vi "Begin.vi"(8 "error in (no error)":errorcluster, 11 "Blocker in":refnum<class "Blocker.lvclass">) -> (0 "error out":errorcluster, 3 "Blocker out":refnum<class "Blocker.lvclass">)   [LabVIEW 2013, in "Blocker.lvclass"]
uses:
  Blocker.lvclass
  <vilib>/Rock Robotics/WPI/Solenoid/WPI_SolenoidChannel.ctl
  <vilib>/Rock Robotics/SystemInterfaces/Typedef/FPGA_TypedefSolenoidModule.ctl
  System/System.lvclass
  <vilib>/Rock Robotics/WPI/Solenoid/WPI_SolenoidOpenSingle.vi
panel:
  in  "Solenoid Module (Module 1)":T1
  in  "Solenoid Channel":T2=enum."Solenoid 5"
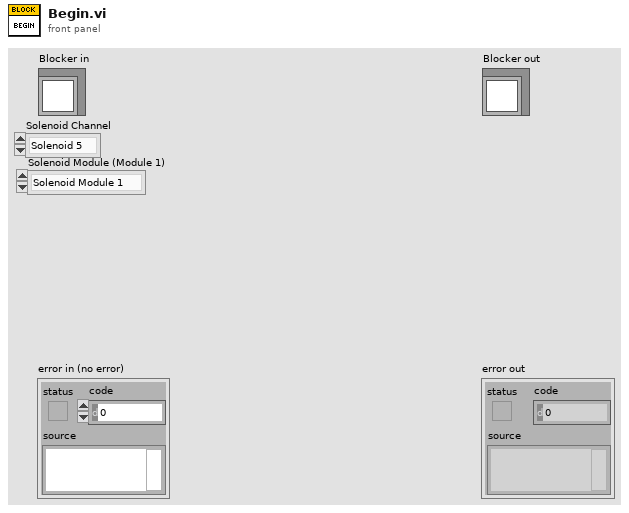
[diagram p1: front panel]
types:
  T1 = typedef "FPGA_TypedefSolenoidModule.ctl" = enum16{"Solenoid Module 1", "Solenoid Module 2"}
  T2 = typedef "WPI_SolenoidChannel.ctl" = enum8{"Solenoid 1", "Solenoid 2", "Solenoid 3", "Solenoid 4", "Solenoid 5", "Solenoid 6", "Solenoid 7", "Solenoid 8", "Invalid"}
  T3 = typedef "WPI_SolenoidDevRef.ctl" = cluster{"DevStatus":errorcluster, "Solenoid Module":T1, "Forward Solenoid Channel":T2, "Reverse Solenoid Channel":T2}
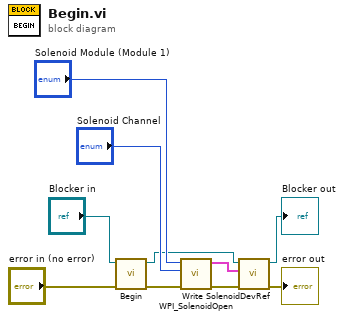
[diagram p0: block diagram]
diagram:
  n1 = call-parent "Begin.vi"("error in (no error)"="error in (no error)", "System in"="Blocker in") -> ("error out"=w2:errorcluster, "System out"=w5:refnum<class "Blocker.lvclass">)  [unwired: 8 in]
  n2 = call-poly <vilib>:"WPI_SolenoidOpen.vi"("error in (no error)"=w2, "Solenoid Channel"="Solenoid Channel", "Solenoid Module (Module 1)"="Solenoid Module (Module 1)") -> ("error out"=w1:errorcluster, "SolenoidDevRef"=w3:T3)  [unwired: 7 in]
  n3 = call-dynamic "Write SolenoidDevRef.vi"("error in (no error)"=w1, "SolenoidDevRef"=w3, "Blocker in"=w5) -> ("error out"=→"error out":errorcluster, "Blocker out"=→"Blocker out":refnum<class "Blocker.lvclass">)  [unwired: 7 in]
